vi "S2C_M2p5942_Proc_Mode.vi"(7 "Local?":bool, 8 "Error In":errorcluster, 10 "Command":string, 11 "JSON String":string) -> (0 "Error Out":errorcluster, 3 "Response":variant)   [LabVIEW 2024]
uses:
  S2C_M2p5942_Proc_Globals.vi
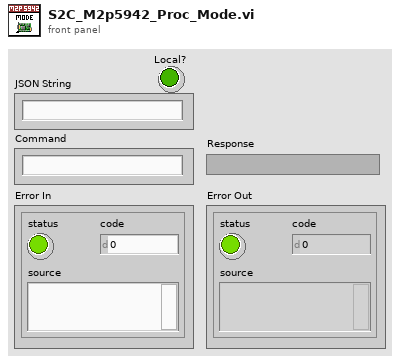
[diagram p1: front panel]
types:
  T1 = cluster{"Mode":u16, "Memory":u32, "Segment Size":u32, "PostTrigger":u32, "PreTrigger":u32, "ABA Mode":u32}
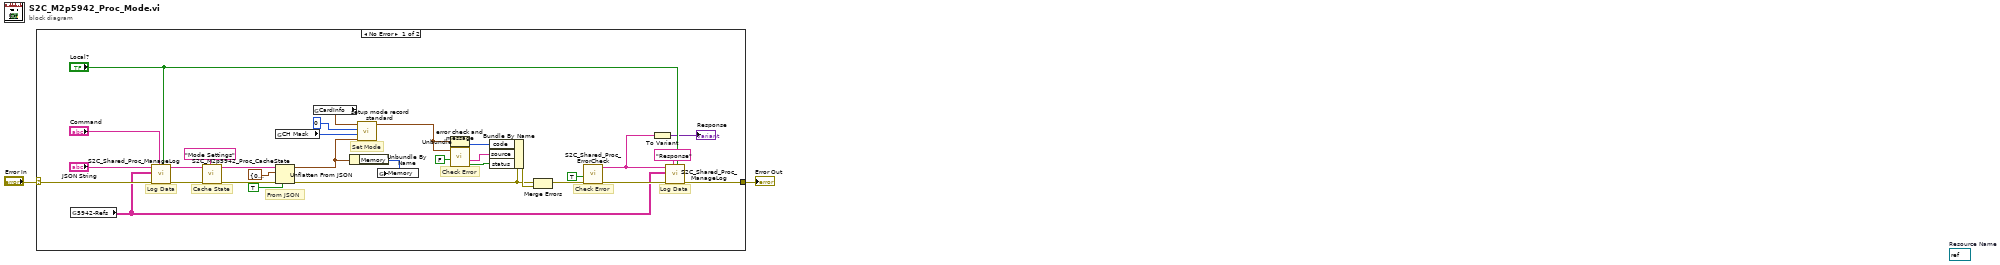
[diagram p0: block diagram]
diagram:
  (unwired) refnum<visa-resource-name> refnum  # Resource Name
  n1 = case shown="No Error" "Error In" {
    selector: "Error In" -> [w32 w34]
    tunnel: [w30 w34] -> w1
    frame No Error {
      # "Check Error"
      # "Set Mode"
      # "Check Error"
      # "Cache State"
      # "Log Data"
      # "Log Data"
      # "From JSON"
      n2 = global read "S2C_M2p5942_Proc_Globals.vi" "5942-Refs"() -> (w20:string[][])
      n3 = call "S2C_Shared_Proc_ManageLog.vi"("Local?"="Local?", "Command"="Command", "Error In"=w32, "Refs"=w20, "Data In"="JSON String") -> ("Error Out"=w28:errorcluster, "Data Out"=w27:string)  [unwired: 5 in]
      n4 = call "S2C_M2p5942_Proc_CacheState.vi"("Label"="Mode Settings", "Error In"=w28, "Data In"=w27) -> ("Error Out"=w25:errorcluster, "Data Out"=w26:string)  [unwired: 7 in]
      n5 = Unflatten From JSON(JSON string=w26, type and defaults=T1 {"Mode"=0, "Memory"=16384, "Segment Size"=1024, "PostTrigger"=8192, "PreTrigger"=32, "ABA Mode"=16} ("Mode Settings"), default null elements? (F)=TRUE, error in (no error)=w25) -> (value=w12:T1, error out=w5:errorcluster)  [unwired: 3 in]
      n6 = global read "S2C_M2p5942_Proc_Globals.vi" "CH Mask"() -> (w15:u32)
      n7 = global read "S2C_M2p5942_Proc_Globals.vi" "CardInfo"() -> (w17:cluster{"Card Handle":u64, "Error Code":u32})
      n8 = Unbundle By Name(w12) -> ("Memory"=w11:u32)
      n9 = call "setup mode record standard.vi"("Mode Setup"=w12, "Channel Mask Low"=w15, "Channel Mask High"=u32 0, "Card Info In"=w17) -> ("Card Info Out"=w4:cluster{"Card Handle":u64, "Error Code":u32})  [unwired: 2 in, 1 out]
      n10 = global write "S2C_M2p5942_Proc_Globals.vi" "Memory"(w11) -> ()
      n11 = Unbundle(w4) -> ("Error Code"=w8:u32)  [unwired: 1 out]
      n12 = call "error check and message.vi"("Display Message (true)"=FALSE, "Card Info In"=w4) -> ("Error occurred"=w6:bool, "Error Message"=w7:string)  [unwired: 3 in, 1 out]
      n13 = Bundle By Name(cluster=w5, "code"=w8, "source"=w7, "status"=w6) -> (w10:errorcluster)
      n14 = Merge Errors(w5, w10) -> (w3:errorcluster)
      n15 = call "S2C_Shared_Proc_ErrorCheck.vi"("Error In"=w3, "ExpReply?"=TRUE) -> ("Error Out"=w22:errorcluster, "Status"=w18:string)  [unwired: 8 in]
      n16 = To Variant(anything=w18) -> (Variant=→"Response":variant)
      n17 = call "S2C_Shared_Proc_ManageLog.vi"("Local?"="Local?", "Command"="Response", "Error In"=w22, "Refs"=w20, "Data In"=w18) -> ("Error Out"=w30:errorcluster)  [unwired: 5 in, 1 out]
    }
    frame Error {
    }
  }
  "Error Out" <- w1
